vi "Switch Output Channel.vi"(8 "error in (no error)":errorcluster, 9 "New Channel":u8, 10 "Old Channel":u8, 11 "QCS in":refnum<class "QCS.lvclass">) -> (0 "error out":errorcluster, 3 "QCS out":refnum<class "QCS.lvclass">)   [LabVIEW 2013, in "QCS.lvclass"]
uses:
  Lib.llb/QCS.lvclass
  Lib.llb/CS.lvclass
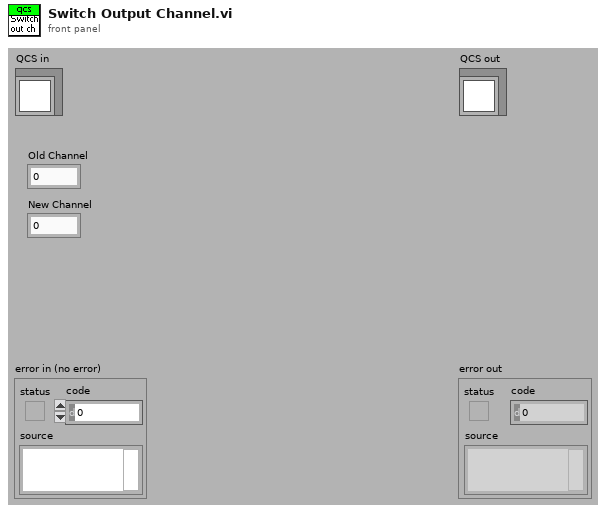
[diagram p1: front panel]
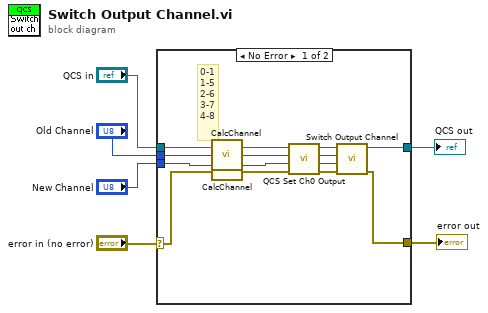
[diagram p0: block diagram]
diagram:
  n1 = case shown="No Error" "error in (no error)" {
    selector: "error in (no error)" -> [w16 w20]
    tunnel: [w11 w20] -> w6
    tunnel: [w18 w19] -> w1
    tunnel: "New Channel" -> [w8 _]
    tunnel: "Old Channel" -> [w10 _]
    tunnel: "QCS in" -> [w15 w19]
    frame No Error {
      # "0-1\n1-5\n2-6\n3-7\n4-8"
      n2 = call "CalcChannel.vi"("Old Channel"=w10) -> ("Numeric"=w9:u8)
      n3 = call "CalcChannel.vi"("Old Channel"=w8) -> ("Numeric"=w7:u8)
      n4 = call "QCS Set Ch0 Output.vi"("error IO"=w16, "New Channel"=w7, "Old Channel"=w9, "QCS in"=w15) -> ("error out"=w17:errorcluster, "Channel"=w12:i32, "OldChannel"=w13:i32, "QCS out"=w14:refnum<class "QCS.lvclass">)
      n5 = call-parent "Switch Output Channel.vi"("error in (no error)"=w17, "New Channel"=w12, "Old Channel"=w13, "CS in"=w14) -> ("error out"=w11:errorcluster, "CS out"=w18:refnum<class "QCS.lvclass">)  [unwired: 6 in]
    }
    frame Error {
    }
  }
  "error out" <- w6
  "QCS out" <- w1
